vi "GetDLLDirectory.vi"(8 "error in (no error)":errorcluster, 10 "DLLDirectoryName":string="EC-Lab Development Package", 11 "AppParentDirectory":path) -> (0 "error out":errorcluster, 2 "DLLDirectory":path, 3 "DLLDirectoryFound":bool)   [LabVIEW 2022 SP3, in "EClib functions.lvlib"]
uses:
  EClib functions.lvlib
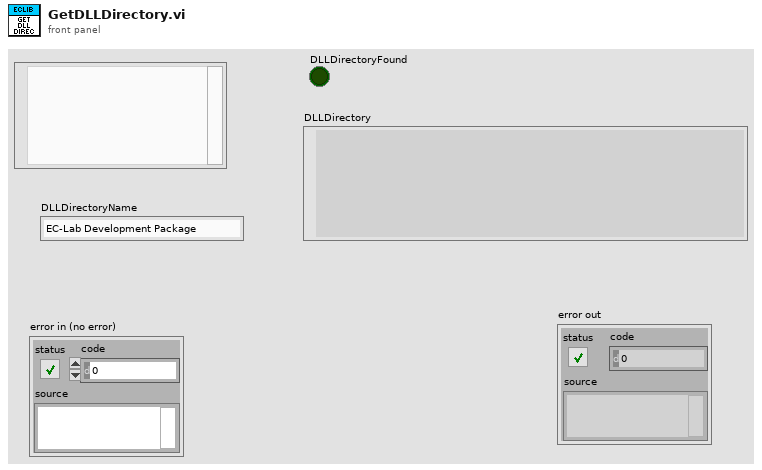
[diagram p1: front panel]
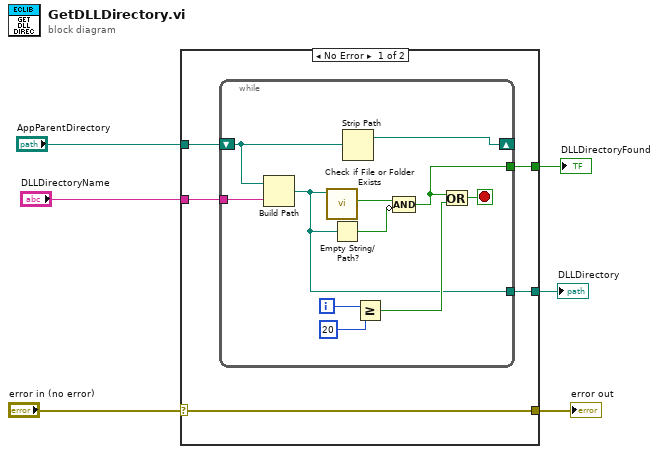
[diagram p0: block diagram]
diagram:
  n1 = case shown="No Error" "error in (no error)" {
    selector: "error in (no error)" -> [w7 w23]
    tunnel: "AppParentDirectory" -> [w11 _]
    tunnel: [w10 _] -> w5
    tunnel: "DLLDirectoryName" -> [w9 _]
    tunnel: [w8 _] -> w3
    tunnel: [w7 w23] -> w1
    frame No Error {
      n2 = while {
        shift-right: [w22] -> _
        shift-left: w11 -> [w16]
        tunnel: [w13] -> w10
        tunnel: w9 -> [w17]
        tunnel: [w14] -> w8
        i -> [w21]
        stop <- w19 stop-if-true
        n3 = Build Path(base path=w16, name or relative path=w17) -> (appended path=w13:path)
        n4 = call <vilib>:"Check if File or Folder Exists.vi"("path"=w13) -> ("file or folder exists?"=w15:bool)  [unwired: 8 in, 2 out]
        n5 = Empty String/Path?(string/path=w13) -> (empty?=w12:bool)
        n6 = Strip Path(path=w16) -> (stripped path=w22:path)  [unwired: 1 out]
        n7 = Greater Or Equal?(x=w21, y=20) -> (x >= y?=w18:bool)
        n8 = Compound Arithmetic op=AND(w15, invert w12) -> (w14:bool)
        n9 = Or(x=w14, y=w18) -> (x .or. y?=w19:bool)
      }
    }
    frame Error {
    }
  }
  "DLLDirectory" <- w5
  "DLLDirectoryFound" <- w3
  "error out" <- w1
